vi "Co-Pilot Log Write.vi"(8 "drive log":refnum<file>, 9 "Co-Pilot Data":T1) -> ()   [LabVIEW 2014]
uses:
  Co-Pilot_game_control.ctl
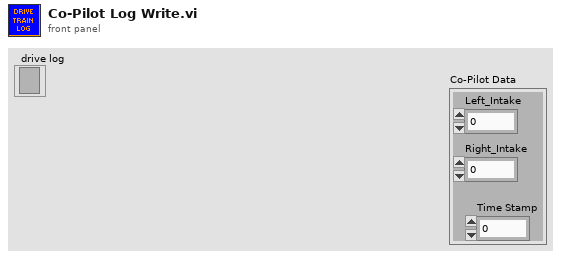
[diagram p1: front panel]
types:
  T1 = typedef "Co-Pilot_game_control.ctl" = cluster{"Left_Intake":dbl, "Right_Intake":dbl, "Time Stamp":dbl}
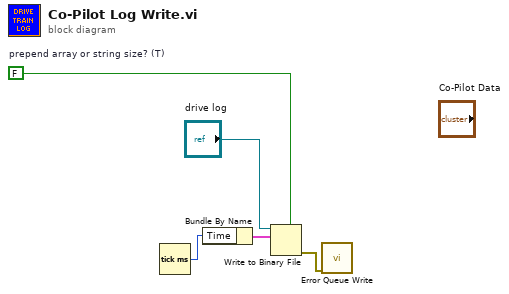
[diagram p0: block diagram]
diagram:
  w2 = FALSE  # prepend array or string size? (T)
  n1 = Tick Count (ms)() -> (millisecond timer value=w5:u32)
  n2 = Bundle By Name("Time"=w5) -> (w4:cluster{}, w6:cluster{})
  n3 = Write to Binary File(file (use dialog)="drive log", data=w4, 5:w2) -> (error out=w1:errorcluster)  [unwired: 3 in, 2 out]
  n4 = call "Error Queue Write.vi"("error in (no error)"=w1) -> ()  [unwired: 11 in]
